vi "dashboard.vi"(2 "Array - String":string[](array[string])) -> (13 "total":i32, 14 "SERVICABLE":i32, 15 "SCRAP":i32, 16 "USED":i32, 17 "RESERVED":i32, 18 "REPAIR":i32, 19 "CALIBRATION":i32)   [LabVIEW 2018]
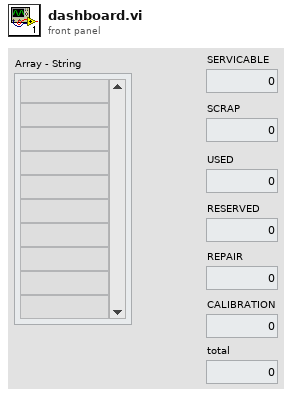
[diagram p1: front panel]
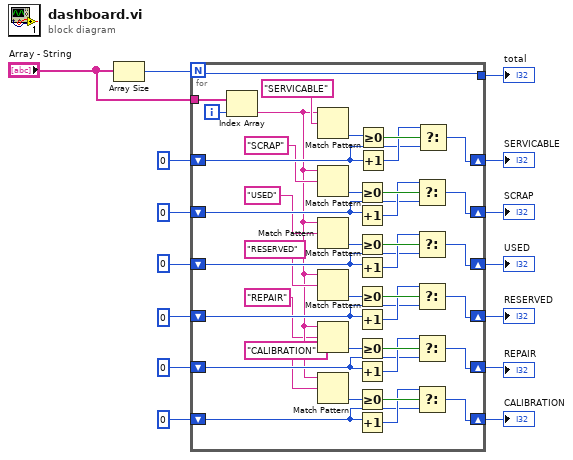
[diagram p0: block diagram]
diagram:
  n1 = Array Size(array="Array - String") -> (size(s)=w15:i32)
  n2 = for {
    N: w15 -> [w55]
    tunnel: "Array - String" -> [w54]
    tunnel: [w55] -> w13
    shift-right: [w47] -> w11
    shift-left: 0 -> [w48]
    shift-right: [w41] -> w9
    shift-left: 0 -> [w42]
    shift-right: [w36] -> w7
    shift-left: 0 -> [w37]
    shift-right: [w29] -> w5
    shift-left: 0 -> [w30]
    shift-right: [w24] -> w3
    shift-left: 0 -> [w25]
    shift-right: [w19] -> w1
    shift-left: 0 -> [w20]
    i -> [w53]
    n3 = Index Array(array=w54, index=w53) -> (element=w18:string)
    n4 = Match Pattern(string=w18, regular expression="SERVICABLE") -> (offset past match=w51:i32)  [unwired: 1 in, 3 out]
    n5 = Match Pattern(string=w18, regular expression="SCRAP") -> (offset past match=w43:i32)  [unwired: 1 in, 3 out]
    n6 = Match Pattern(string=w18, regular expression="USED") -> (offset past match=w38:i32)  [unwired: 1 in, 3 out]
    n7 = Match Pattern(string=w18, regular expression="RESERVED") -> (offset past match=w32:i32)  [unwired: 1 in, 3 out]
    n8 = Match Pattern(string=w18, regular expression="REPAIR") -> (offset past match=w26:i32)  [unwired: 1 in, 3 out]
    n9 = Match Pattern(string=w18, regular expression="CALIBRATION") -> (offset past match=w21:i32)  [unwired: 1 in, 3 out]
    n10 = Greater Or Equal To 0?(x=w43) -> (x >= 0?=w45:bool)
    n11 = Increment(x=w42) -> (x+1=w44:i32)
    n12 = Greater Or Equal To 0?(x=w38) -> (x >= 0?=w40:bool)
    n13 = Increment(x=w37) -> (x+1=w39:i32)
    n14 = Greater Or Equal To 0?(x=w32) -> (x >= 0?=w34:bool)
    n15 = Increment(x=w30) -> (x+1=w33:i32)
    n16 = Greater Or Equal To 0?(x=w26) -> (x >= 0?=w28:bool)
    n17 = Increment(x=w25) -> (x+1=w27:i32)
    n18 = Greater Or Equal To 0?(x=w21) -> (x >= 0?=w23:bool)
    n19 = Increment(x=w20) -> (x+1=w22:i32)
    n20 = Greater Or Equal To 0?(x=w51) -> (x >= 0?=w50:bool)
    n21 = Increment(x=w48) -> (x+1=w49:i32)
    n22 = Select(t=w44, s=w45, f=w42) -> (s? t:f=w41:i32)
    n23 = Select(t=w39, s=w40, f=w37) -> (s? t:f=w36:i32)
    n24 = Select(t=w33, s=w34, f=w30) -> (s? t:f=w29:i32)
    n25 = Select(t=w27, s=w28, f=w25) -> (s? t:f=w24:i32)
    n26 = Select(t=w22, s=w23, f=w20) -> (s? t:f=w19:i32)
    n27 = Select(t=w49, s=w50, f=w48) -> (s? t:f=w47:i32)
  }
  "SERVICABLE" <- w11
  "USED" <- w7
  "SCRAP" <- w9
  "total" <- w13
  "RESERVED" <- w5
  "REPAIR" <- w3
  "CALIBRATION" <- w1
